vi "Decimal_to_binary.vi"() -> ()   [LabVIEW 2019]
panel:
  in  "Zero":bool
  in  "Stop":bool
  out "Liczba binarnie":bool[](array[boolean])
  in  "Liczba":i8
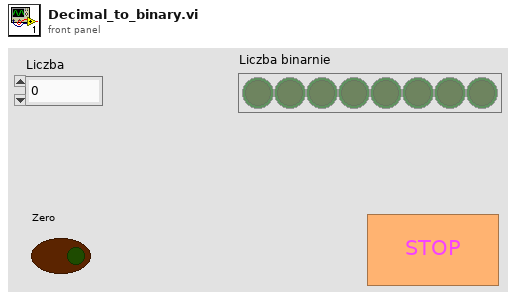
[diagram p1: front panel]
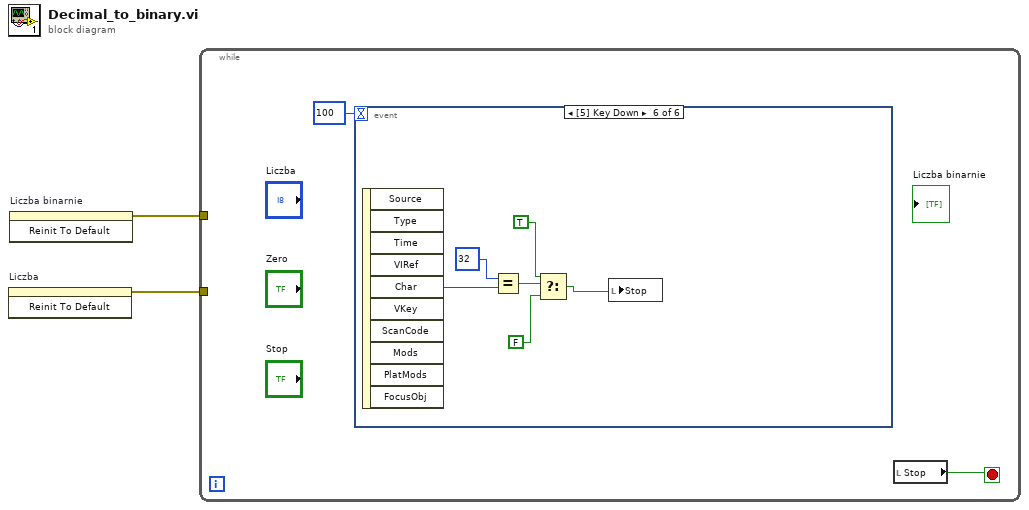
[diagram p0: block diagram]
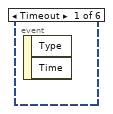
[diagram p2: hidden frame]
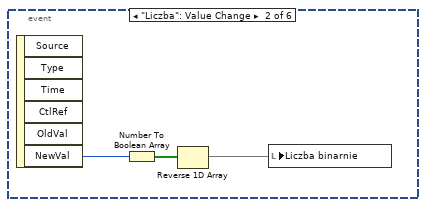
[diagram p3: hidden frame]
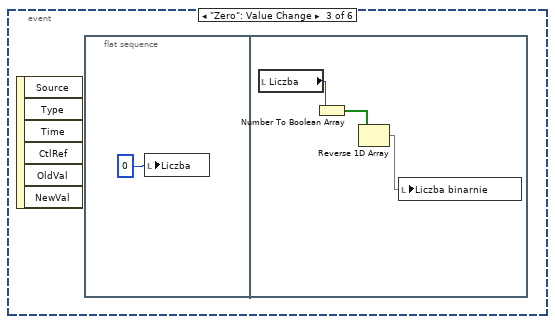
[diagram p4: hidden frame]
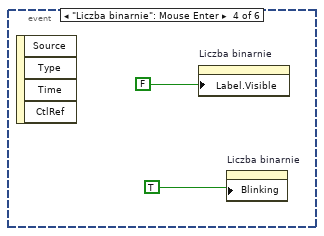
[diagram p5: hidden frame]
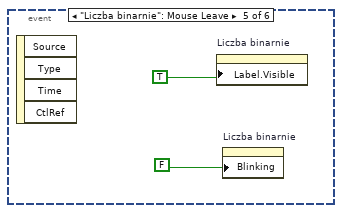
[diagram p6: hidden frame]
diagram:
  n1 = invoke on="Liczba" class="DigNum (strict)" method="Reinit To Default"() -> (error out=w1:errorcluster)  [unwired: 3 in, 2 out]
  n2 = invoke on="Liczba binarnie" class="Arr (strict)" method="Reinit To Default"() -> (error out=w2:errorcluster)  [unwired: 3 in, 2 out]
  n3 = while {
    tunnel: w2 -> [_]
    tunnel: w1 -> [_]
    stop <- w3 stop-if-true
    n4 = event shown="[5] Key Down" {
      selector: _ -> [_ _ _ _ _ _]
      dyn-events: _ -> [_ _ _ _ _ _]
      timeout: 100 -> [_ _ _ _ _ _]
      event Timeout {
        n5 = event-data() -> ()  [unwired: 1 in, 2 out]
      }
      event "Liczba": Value Change {
        n6 = event-data() -> ("NewVal"=w7:i8)  [unwired: 1 in, 5 out]
        n7 = Number To Boolean Array(number=w7) -> (Boolean array=w6:bool[])
        n8 = Reverse 1D Array(array=w6) -> (reversed array=w5:bool[])
        n9 = local write "Liczba binarnie"(w5) -> ()
      }
      event "Zero": Value Change {
        n10 = event-data() -> ()  [unwired: 1 in, 6 out]
        n11 = flat-sequence {
          frame #0 {
            n12 = local write "Liczba"(i8 0 ("Liczba")) -> ()
          }
          frame #1 {
            n13 = local read "Liczba"() -> (w10:i8)
            n14 = Number To Boolean Array(number=w10) -> (Boolean array=w11:bool[])
            n15 = Reverse 1D Array(array=w11) -> (reversed array=w9:bool[])
            n16 = local write "Liczba binarnie"(w9) -> ()
          }
        }
      }
      event "Liczba binarnie": Mouse Enter {
        n17 = event-data() -> ()  [unwired: 1 in, 4 out]
        n18 = property on="Liczba binarnie" class="Arr (strict)"("Label.Visible"=FALSE) -> ()  [unwired: 2 in, 2 out]
        n19 = property on="Liczba binarnie" class="Arr (strict)"("Blinking"=TRUE) -> ()  [unwired: 2 in, 2 out]
      }
      event "Liczba binarnie": Mouse Leave {
        n20 = event-data() -> ()  [unwired: 1 in, 4 out]
        n21 = property on="Liczba binarnie" class="Arr (strict)"("Label.Visible"=TRUE) -> ()  [unwired: 2 in, 2 out]
        n22 = property on="Liczba binarnie" class="Arr (strict)"("Blinking"=FALSE) -> ()  [unwired: 2 in, 2 out]
      }
      event Key Down {
        n23 = event-data() -> ("Char"=w20:i16)  [unwired: 1 in, 9 out]
        n24 = Equal?(x=i16 32 ("y"), y=w20) -> (x = y?=w19:bool)
        n25 = Select(t=TRUE, s=w19, f=FALSE) -> (s? t:f=w16:bool)
        n26 = local write "Stop"(w16) -> ()
      }
    }
    n27 = local read "Stop"() -> (w3:bool)
  }
